vi "Script VIs.vi"(6 "VI Refs":T5, 8 "error in":errorcluster, 9 "Msg Output Terminal Map":T1, 10 "Msg Terminal Map":T3) -> (0 "error out":errorcluster)   [LabVIEW 2025, in "_Msg Rescript.lvlib" / "_Msg Rescript.lvclass"]
uses:
  _Msg Rescript.lvclass
  _Msg Rescript.lvclass/_Msg Rescript.ctl
  <vilib>/Utility/traverseref.llb/TRef TravTarget.ctl
  VI Refs.ctl
  Msg Terminal Attributes.ctl
  Msg Terminal Map.ctl
  Msg Output Terminal Attributes.ctl
  Msg Output Terminal Map.ctl
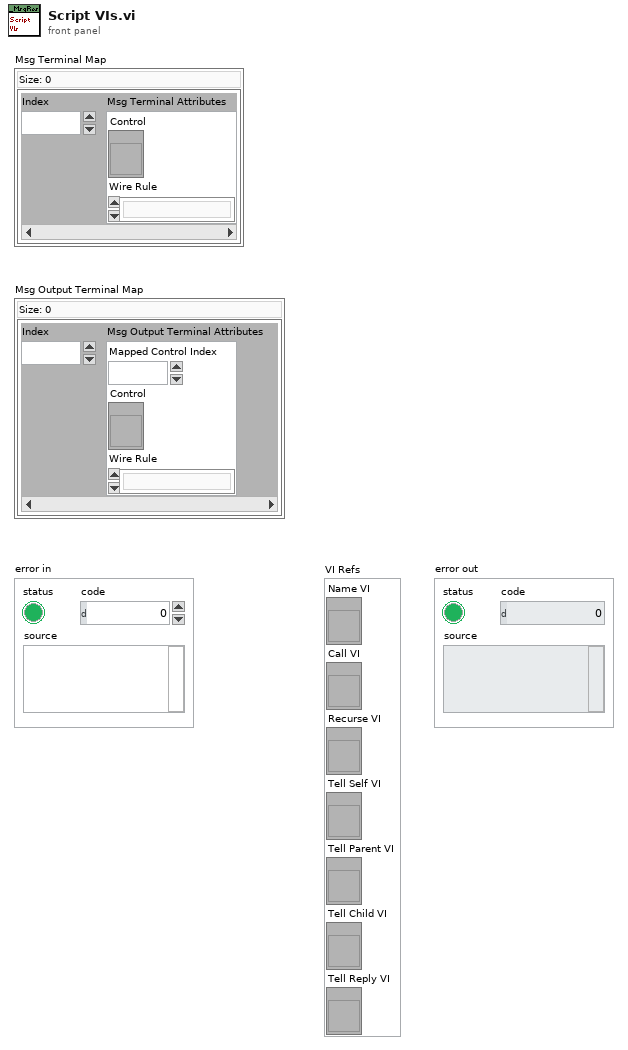
[diagram p1: front panel]
types:
  T1 = typedef "_Msg Rescript.lvlib/_Msg Rescript.lvclass/Msg Output Terminal Map.ctl" = map{i32, T2}
  T2 = typedef "_Msg Rescript.lvlib/_Msg Rescript.lvclass/Msg Output Terminal Attributes.ctl" = cluster{"Mapped Control Index":i32, "Control":refnum<vi>, "Wire Rule":enum16{"Invalid Wire Rule", "Required", "Recommended", "Optional", "Dynamic Dispatch"}}
  T3 = typedef "_Msg Rescript.lvlib/_Msg Rescript.lvclass/Msg Terminal Map.ctl" = map{i32, T4}
  T4 = typedef "_Msg Rescript.lvlib/_Msg Rescript.lvclass/Msg Terminal Attributes.ctl" = cluster{"Control":refnum<vi>, "Wire Rule":enum16{"Invalid Wire Rule", "Required", "Recommended", "Optional", "Dynamic Dispatch"}}
  T5 = typedef "_Msg Rescript.lvlib/_Msg Rescript.lvclass/VI Refs.ctl" = cluster{"Name VI":refnum<vi>, "Call VI":refnum<vi>, "Recurse VI":refnum<vi>, "Tell Self VI":refnum<vi>, "Tell Parent VI":refnum<vi>, "Tell Child VI":refnum<vi>, "Tell Reply VI":refnum<vi>}
  T6 = typedef "TRef TravTarget.ctl" = enum16{"FP", "BD", "Other"}
  T7 = enum16{"Invalid Wire Rule", "Required", "Recommended", "Optional", "Dynamic Dispatch"}
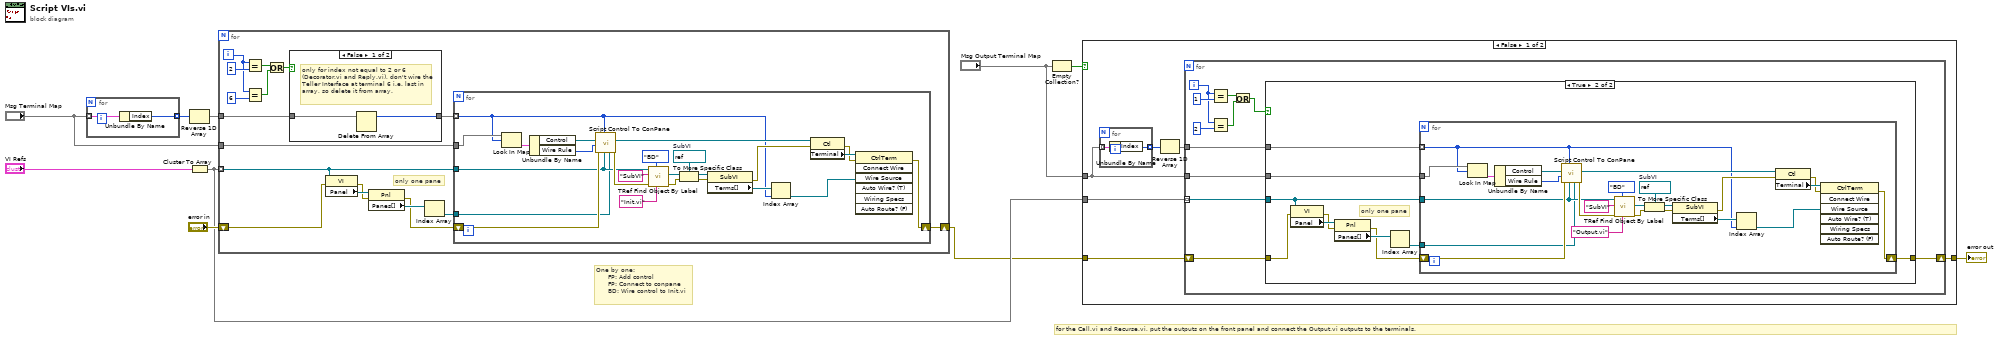
[diagram p0: block diagram]
diagram:
  # "for the Call.vi and Recurse.vi, put the outputs on the front panel and connect the Output.vi outputs to the terminals."
  # "One by one:\n      FP: Add control\n      FP: Connect to conpane\n      BD: Wire control to Init.vi"
  n1 = for {
    tunnel: "Msg Terminal Map" -> [w12] mode=indexing
    tunnel: [w11] -> w10 mode=indexing
    n2 = Unbundle By Name(w12) -> ("Index"=w11:i32)
  }
  n3 = Reverse 1D Array(array=w10) -> (reversed array=w9:i32[])
  n4 = Cluster To Array(cluster="VI Refs") -> (array=w4:refnum<vi>[])
  n5 = for {
    tunnel: w9 -> [w19]
    tunnel: "Msg Terminal Map" -> [w29]
    shift-right: [w27] -> w2
    shift-left: "error in" -> [w28]
    tunnel: w4 -> [w25] mode=indexing
    i -> [w13]
    # "only one pane"
    n6 = Equal?(x=w13, y=2) -> (x = y?=w17:bool)
    n7 = Equal?(x=w13, y=6) -> (x = y?=w14:bool)
    n8 = Or(x=w17, y=w14) -> (x .or. y?=w16:bool)
    n9 = case shown="False" w16 {
      tunnel: w19 -> [w31 w32]
      tunnel: [w30 w32] -> w18
      frame False {
        # "only for index not equal to 2 or 6 (Decorator.vi and Reply.vi), don't wire the Teller Interface at terminal 6 i.e. last in array, so delete it from array."
        n10 = Delete From Array(array=w31) -> (array with subset deleted=w30:i32[])  [unwired: 2 in, 1 out]
      }
      frame True {
      }
    }
    n11 = property class="VI"(reference=w25, error in=w28) -> (error out=w22:errorcluster, "Panel"=w24:refnum<vi>)  [unwired: 1 out]
    n12 = property class="Pnl"(reference=w24, error in=w22) -> (error out=w21:errorcluster, "Panes[]"=w23:refnum<vi>[])  [unwired: 1 out]
    n13 = Index Array(array=w23) -> (element=w20:refnum<vi>)  [unwired: 1 in]
    n14 = for {
      tunnel: w18 -> [w33] mode=indexing
      tunnel: w29 -> [w36]
      tunnel: w20 -> [w38]
      tunnel: w25 -> [w39]
      shift-right: [w54] -> w27
      shift-left: w21 -> [w42]
      w52 = refnum<vi> refnum  # SubVI
      n15 = Look In Map(map=w36, key=w33) -> (value=w37:T4)  [unwired: 1 in, 1 out]
      n16 = Unbundle By Name(w37) -> ("Control"=w35:refnum<vi>, "Wire Rule"=w34:T7)
      n17 = call "Script Control To ConPane.vi"("Pane"=w38, "VI Ref"=w39, "Terminal Index"=w33, "error in"=w42, "Wire Rule"=w34, "Control"=w35) -> ("error out"=w41:errorcluster, "Control"=w40:refnum<vi>)  [unwired: 4 in]
      n18 = call <vilib>:"TRef Find Object By Label.vi"("Label"="Init.vi", "Traverse Target"=TRef_TravTarget."BD", "error in (no error)"=w41, "Class Name"="SubVI", "VI Ref"=w39) -> ("error out"=w51:errorcluster, "Found Obj Ref"=w46:refnum<vi>)  [unwired: 3 in, 2 out]
      n19 = To More Specific Class(target class=w52, reference=w46, error in=w51) -> (specific class reference=w49:refnum<vi>, error out=w48:errorcluster)
      n20 = property class="SubVI"(reference=w49, error in=w48) -> (error out=w43:errorcluster, "Terms[]"=w47:refnum<vi>[])  [unwired: 1 out]
      n21 = Index Array(array=w47, index=w33) -> (element=w44:refnum<vi>)
      n22 = property class="Ctl"(reference=w40, error in=w43) -> (error out=w55:errorcluster, "Terminal"=w56:refnum<vi>)  [unwired: 1 out]
      n23 = invoke class="CtrlTerm" method="Connect Wire"(reference=w56, error in=w55, "Wire Source"=w44) -> (error out=w54:errorcluster)  [unwired: 4 in, 6 out]
    }
  }
  n24 = Empty Collection?(1:"Msg Output Terminal Map") -> (0:w5:bool)
  n25 = case shown="False" w5 {
    tunnel: w4 -> [w62 _]
    tunnel: "Msg Output Terminal Map" -> [w60 _]
    tunnel: w2 -> [w58 w111]
    tunnel: [w57 w111] -> w1
    frame False {
      n26 = for {
        tunnel: w60 -> [w64] mode=indexing
        tunnel: [w63] -> w61 mode=indexing
        n27 = Unbundle By Name(w64) -> ("Index"=w63:i32)
      }
      n28 = Reverse 1D Array(array=w61) -> (reversed array=w59:i32[])
      n29 = for {
        tunnel: w59 -> [w66]
        tunnel: w60 -> [w75]
        shift-right: [w73] -> w57
        shift-left: w58 -> [w74]
        tunnel: w62 -> [w71] mode=indexing
        i -> [w67]
        n30 = Equal?(x=w67, y=1) -> (x = y?=w70:bool)
        n31 = Equal?(x=w67, y=2) -> (x = y?=w68:bool)
        n32 = Or(x=w70, y=w68) -> (x .or. y?=w65:bool)
        n33 = case shown="True" w65 {
          tunnel: w75 -> [_ w86]
          tunnel: w74 -> [w76 w85]
          tunnel: [w76 w84] -> w73
          tunnel: w71 -> [_ w83]
          tunnel: w66 -> [_ w77]
          frame False {
          }
          frame True {
            # "only one pane"
            n34 = property class="VI"(reference=w83, error in=w85) -> (error out=w80:errorcluster, "Panel"=w82:refnum<vi>)  [unwired: 1 out]
            n35 = property class="Pnl"(reference=w82, error in=w80) -> (error out=w79:errorcluster, "Panes[]"=w81:refnum<vi>[])  [unwired: 1 out]
            n36 = Index Array(array=w81) -> (element=w78:refnum<vi>)  [unwired: 1 in]
            n37 = for {
              tunnel: w77 -> [w87] mode=indexing
              tunnel: w86 -> [w90]
              tunnel: w78 -> [w92]
              tunnel: w83 -> [w93]
              shift-right: [w108] -> w84
              shift-left: w79 -> [w96]
              w106 = refnum<vi> refnum  # SubVI
              n38 = Look In Map(map=w90, key=w87) -> (value=w91:T2)  [unwired: 1 in, 1 out]
              n39 = Unbundle By Name(w91) -> ("Control"=w89:refnum<vi>, "Wire Rule"=w88:T7)
              n40 = call "Script Control To ConPane.vi"("Pane"=w92, "VI Ref"=w93, "Terminal Index"=w87, "error in"=w96, "Wire Rule"=w88, "Control"=w89) -> ("error out"=w95:errorcluster, "Control"=w94:refnum<vi>)  [unwired: 4 in]
              n41 = call <vilib>:"TRef Find Object By Label.vi"("Label"="Output.vi", "Traverse Target"=TRef_TravTarget."BD", "error in (no error)"=w95, "Class Name"="SubVI", "VI Ref"=w93) -> ("error out"=w105:errorcluster, "Found Obj Ref"=w100:refnum<vi>)  [unwired: 3 in, 2 out]
              n42 = To More Specific Class(target class=w106, reference=w100, error in=w105) -> (specific class reference=w103:refnum<vi>, error out=w102:errorcluster)
              n43 = property class="SubVI"(reference=w103, error in=w102) -> (error out=w97:errorcluster, "Terms[]"=w101:refnum<vi>[])  [unwired: 1 out]
              n44 = Index Array(array=w101, index=w87) -> (element=w98:refnum<vi>)
              n45 = property class="Ctl"(reference=w94, error in=w97) -> (error out=w109:errorcluster, "Terminal"=w110:refnum<vi>)  [unwired: 1 out]
              n46 = invoke class="CtrlTerm" method="Connect Wire"(reference=w110, error in=w109, "Wire Source"=w98) -> (error out=w108:errorcluster)  [unwired: 4 in, 6 out]
            }
          }
        }
      }
    }
    frame True {
    }
  }
  "error out" <- w1
